vi "Get DefinedName.vi"(7 "Sheet Name":string, 8 "error in":errorcluster, 10 "Range Identifier":string, 11 "SpreadsheetDoc in":refnum<k24>) -> (0 "error out":errorcluster, 2 "DefinedName":refnum<k24>, 3 "SpreadsheetDoc out":refnum<k24>, 5 "Sheet Name":string)   [LabVIEW 2019, in "Open Xml.lvlib"]
uses:
  Open Xml.lvlib
  D:/git/Open-Xml-LabVIEW/Source/DocumentFormat.OpenXml.dll
  DocumentFormat.OpenXml.dll
  D:/git/Open-Xml-LabVIEW/Source/DocumentFormat.OpenXml.Framework.dll
  DocumentFormat.OpenXml.Framework.dll
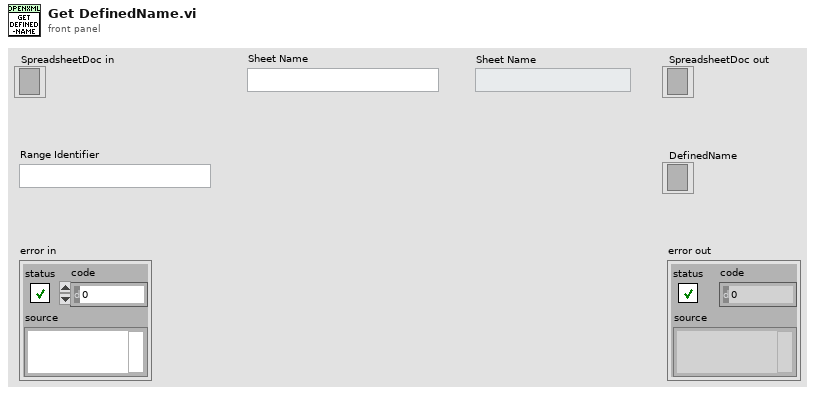
[diagram p1: front panel]
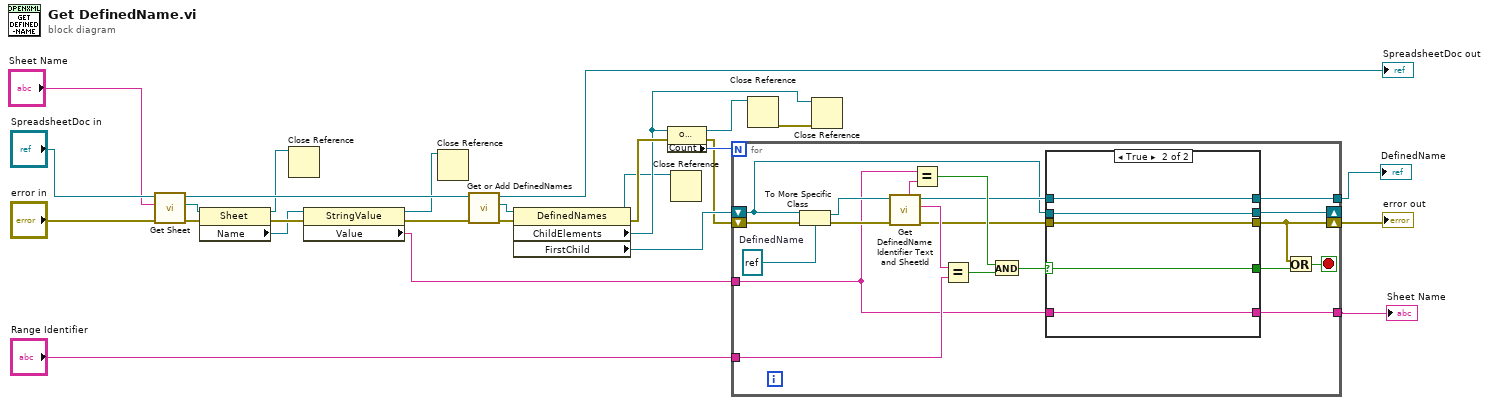
[diagram p0: block diagram]
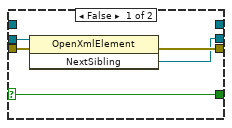
[diagram p2: hidden frame]
diagram:
  n1 = call "Get Sheet.vi"("error in"="error in", "SheetName"="Sheet Name", "SpreadsheetDoc in"="SpreadsheetDoc in") -> ("error out"=w16:errorcluster, "Sheet"=w11:refnum<k24>, "SpreadsheetDoc out"=w14:refnum<k24>)  [unwired: 5 in, 1 out]
  n2 = property class="Sheet"(reference=w11, error in=w16) -> (reference out=w8:refnum<k24>, error out=w12:errorcluster, "Name"=w9:refnum<k24>)
  n3 = Close Reference(reference=w8) -> ()  [unwired: 1 in, 1 out]
  n4 = property class="StringValue"(reference=w9, error in=w12) -> (reference out=w7:refnum<k24>, error out=w10:errorcluster, "Value"=w2:string)
  n5 = Close Reference(reference=w7) -> ()  [unwired: 1 in, 1 out]
  n6 = call "Get or Add DefinedNames.vi"("error in"=w10, "SpreadsheetDoc in"=w14) -> ("error out"=w26:errorcluster, "DefinedNames"=w25:refnum<k24>, "SpreadsheetDoc out"=→"SpreadsheetDoc out":refnum<k24>)  [unwired: 7 in]
  n7 = property class="DefinedNames"(reference=w25, error in=w26) -> (reference out=w5:refnum<k24>, error out=w23:errorcluster, "ChildElements"=w19:refnum<k24>, "FirstChild"=w22:refnum<k24>)
  n8 = property class="OpenXmlElementList"(reference=w19, error in=w23) -> (reference out=w21:refnum<k24>, error out=w20:errorcluster, "Count"=w24:i32)
  n9 = Close Reference(reference=w5) -> ()  [unwired: 1 in, 1 out]
  n10 = for {
    N: w24 -> [_]
    tunnel: "Range Identifier" -> [w43]
    tunnel: w2 -> [w30]
    shift-right: [w38] -> w6
    shift-left: w20 -> [w47]
    shift-right: [w33] -> _
    shift-left: w22 -> [w34]
    tunnel: [w31] -> w4
    tunnel: [w29] -> w1
    stop <- w40 stop-if-true
    w32 = refnum<k24> refnum  # DefinedName
    n11 = To More Specific Class(target class=w32, reference=w34, error in=w47) -> (specific class reference=w35:refnum<k24>, error out=w46:errorcluster)
    n12 = call "Get DefinedName Identifier Text and SheetId.vi"("error in"=w46, "DefinedName in"=w35) -> ("error out"=w39:errorcluster, "Identifier"=w44:string, "DefinedName out"=w37:refnum<k24>, "Sheet Name"=w45:string)  [unwired: 5 in, 1 out]
    n13 = Equal?(x=w30, y=w45) -> (x = y?=w41:bool)
    n14 = Equal?(x=w44, y=w43) -> (x = y?=w42:bool)
    n15 = And(x=w41, y=w42) -> (x .and. y?=w36:bool)
    n16 = case shown="True" w36 {
      selector: w36 -> [w48 w53]
      tunnel: w39 -> [w52 w56]
      tunnel: [w51 w56] -> w38
      tunnel: w37 -> [_ w57]
      tunnel: [w50 w55] -> w33
      tunnel: w34 -> [w49 w55]
      tunnel: [_ w57] -> w31
      tunnel: w30 -> [_ w54]
      tunnel: [_ w54] -> w29
      tunnel: [w48 w53] -> w28
      frame False {
        n17 = invoke class="OpenXmlElement" method="NextSibling"(reference=w49, error in=w52) -> (error out=w51:errorcluster, "NextSibling"=w50:refnum<k24>)  [unwired: 1 in, 1 out]
      }
      frame True {
      }
    }
    n18 = Or(x=w38, y=w28) -> (x .or. y?=w40:bool)
  }
  "error out" <- w6
  "DefinedName" <- w4
  "Sheet Name" <- w1
  n19 = Close Reference(reference=w21) -> (error out=w18:errorcluster)  [unwired: 1 in]
  n20 = Close Reference(reference=w19, error in (no error)=w18) -> ()  [unwired: 1 out]
